vi "Sub_rescale_freq.vi"(10 "Beam frequency params":T1={"Max frequency"=90.12982157307079, "Min frequency"=50.02668540369471, "Max frequency delta per node"=-1.0, "Max frequency delta per second"=-169.531914893617} {"Max frequency delta per node" format="%0.2f"}, 11 "Freq?":dbl) -> (3 "Freq":dbl)   [LabVIEW 2019]
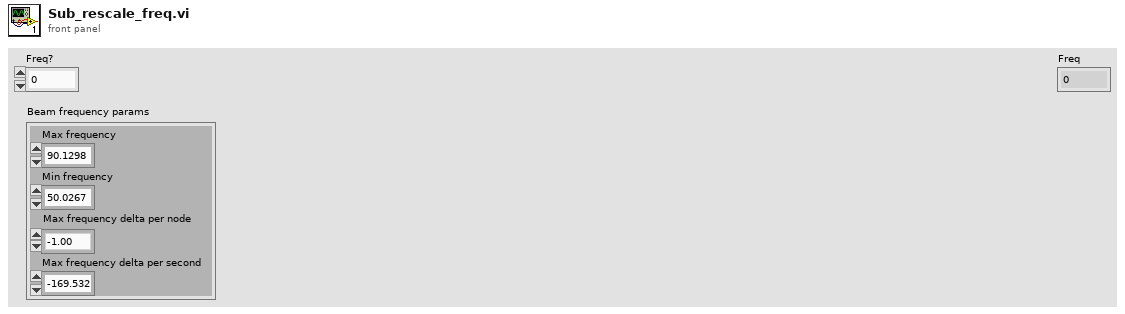
[diagram p1: front panel]
types:
  T1 = cluster{"Max frequency":dbl, "Min frequency":dbl, "Max frequency delta per node":dbl, "Max frequency delta per second":dbl}
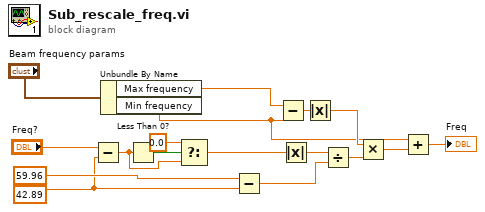
[diagram p0: block diagram]
diagram:
  w15 = 42.89
  n1 = Subtract(x="Freq?", y=w15) -> (x-y=w2:dbl)
  n2 = Unbundle By Name("Beam frequency params") -> ("Max frequency"=w12:dbl, "Min frequency"=w6:dbl)
  n3 = Less Than 0?(x=w2) -> (x < 0?=w4:bool)
  n4 = Select(t=0.0, s=w4, f=w2) -> (s? t:f=w1:dbl)
  n5 = Subtract(x=59.96, y=w15) -> (x-y=w13:dbl)
  n6 = Subtract(x=w12, y=w6) -> (x-y=w11:dbl)
  n7 = Absolute Value(x=w1) -> (abs(x)=w10:dbl)
  n8 = Absolute Value(x=w11) -> (abs(x)=w8:dbl)
  n9 = Divide(x=w10, y=w13) -> (x/y=w9:dbl)
  n10 = Multiply(x=w8, y=w9) -> (x*y=w7:dbl)
  n11 = Add(x=w6, y=w7) -> (x+y=→"Freq":dbl)
